vi "Check Response Bytes.vi"(9 "Data Bytes":u8[](array[numeric]) format="%0x", 11 "Response Bytes":u8[](array[numeric]) format="%0x") -> (3 "Pass?":bool)   [LabVIEW 2018]
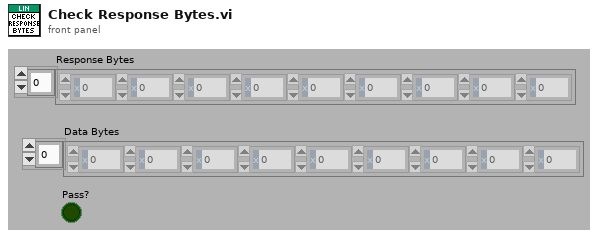
[diagram p1: front panel]
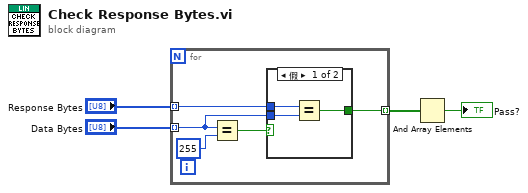
[diagram p0: block diagram]
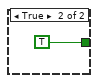
[diagram p2: hidden frame]
diagram:
  n1 = for {
    tunnel: "Response Bytes" -> [w6] mode=indexing
    tunnel: "Data Bytes" -> [w5] mode=indexing
    tunnel: [w7] -> w2 mode=indexing
    n2 = Equal?(x=w5, y=u8 255) -> (x = y?=w8:bool)
    n3 = case shown="假" w8 {
      tunnel: [w10 TRUE] -> w7
      tunnel: w6 -> [w12 _]
      tunnel: w5 -> [w11 _]
      frame False {
        n4 = Equal?(x=w12, y=w11) -> (x = y?=w10:bool)
      }
      frame True {
      }
    }
  }
  n5 = And Array Elements(Boolean array=w2) -> (logical AND=→"Pass?":bool)
